vi "Get Base Command.vi"(8 "error in (no error)":errorcluster, 11 "IDN in":refnum<class "IDN.lvclass">) -> (0 "error out":errorcluster, 2 "Base Command":string, 3 "IDN out":refnum<class "IDN.lvclass">)   [LabVIEW 2023, in "HAF.lvlib" / "IDN.lvclass"]
doc: "Returns the base command whch is used to build up the overall command string – parameters will be added to this as necessary.  The framework will add the line terminator \\n.\n\nSubclasses MUST override this member and must not add a line terminator on the end of the command; on this class an error is returned."
uses:
  IDN.lvclass
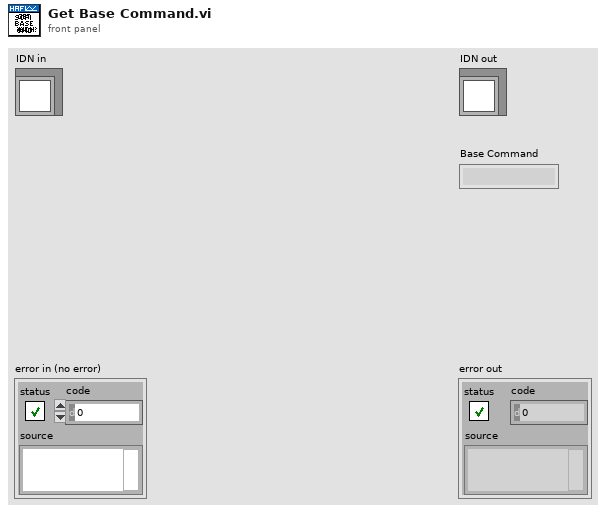
[diagram p1: front panel]
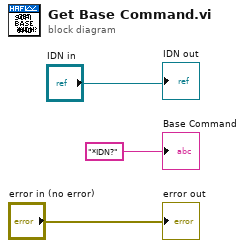
[diagram p0: block diagram]
diagram:
  "error out" <- "error in (no error)"
  "IDN out" <- "IDN in"
  "Base Command" <- "*IDN?" ("Base Command")
